vi "Sub.vi"() -> ()   [LabVIEW 2013, in "User Event Collection.lvclass"]
uses:
  User Event Collection.lvclass
  Method/Tag.ctl
panel:
  in  "UI":dbl
  out "数据":variant
  out "Name":string
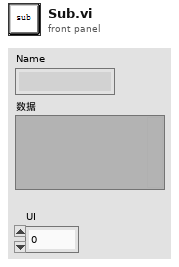
[diagram p1: front panel]
types:
  T1 = enum16{"Init", "Post Event", "Destroy", "Reg Ref"}
  T2 = typedef "User Event Collection.lvclass/Tag.ctl" = enum16{"Main", "UI"}
  T3 = typedef "NISAST Event.lvclass/Event Registeration Refnum.ctl" = refnum<event-registration>
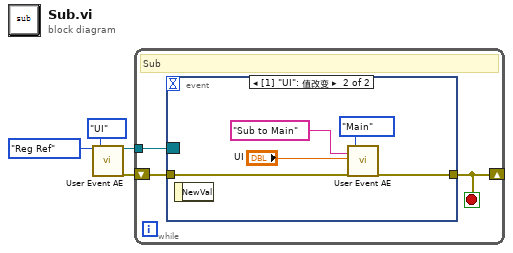
[diagram p0: block diagram]
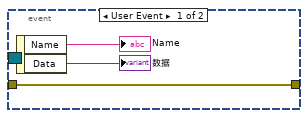
[diagram p2: hidden frame]
diagram:
  n1 = call "User Event AE.vi"("Mode"=T1."Reg Ref", "Tag"=Tag."UI") -> ("Event Registration Refnum"=w1:T3, "error out"=w2:errorcluster)  [unwired: 16 in]
  n2 = while {
    tunnel: w1 -> [w7]
    shift-right: [w5] -> _
    shift-left: w2 -> [w6]
    stop <- w5 stop-if-true
    # "Sub"
    n3 = event shown="[1] \"UI\": 值改变" {
      selector: w7 -> [_ _]
      dyn-events: _ -> [_ _]
      timeout: _ -> [_ _]
      tunnel: w6 -> [w8 w15]
      tunnel: [w8 w14] -> w5
      event User Event {
        n4 = event-data() -> ("Name"=→"Name":string, "Data"=→"数据":variant)  [unwired: 1 in]
      }
      event "UI": Value Change {
        n5 = event-data() -> ()  [unwired: 1 in, 1 out]
        n6 = call "User Event AE.vi"("Event Name"="Sub to Main", "Event Data"="UI", "error in (no error)"=w15, "Tag"=Tag."Main") -> ("error out"=w14:errorcluster)  [unwired: 14 in, 1 out]
      }
    }
  }
